vi "task_Meas.vi"() -> ()   [LabVIEW 2015]
uses:
  Framework/pdbm_test_route/UsrDefine/TaskFeedbackCmd.ctl
  Framework/pdbm_test_route/UsrDefine/TaskReqst.ctl
  <vilib>/DAQmx/read.llb/DAQmx Read (Analog 2D DBL NChan NSamp).vi
  <vilib>/DAQmx/create/channels.llb/DAQmx Create Channel (AI-Voltage-Basic).vi
  <vilib>/DAQmx/configure/timing.llb/DAQmx Timing (Sample Clock).vi
  <vilib>/DAQmx/miscellaneous.llb/DAQmx Fill In Error Info.vi
  Framework/pdbm_tasks/pdbm_tasks.lvlib
  <resource>/objmgr/daqmx.rc
  Framework/pdbm_test_route/pdbm_task_route.lvlib
panel:
  in  "Tab Control":enum32{"Scope", "Spectrum Analyzer"}(tab)
  out "dV":string="142.75 µs" caption="dV:"
  out "Scope graph":dbl[][](graph)=[[-0.0025862696478761516, 0.003794052366753585, -0.011518720468357783, 0.0025179879638276377, -0.01789904248298752, -0.010242656065431836, -0.016622978080061572, -0.008966591662505888, -0.0025862696478761516, 0.003794052366753585, 0.0025179879638276377, -0.0064144628566539935, -0.0013102052449502043, -0.011518720468357783, -0.003862334050802099, -0.008966591662505888, -0.003862334050802099, -0.0064144628566539935, -0.015346913677135626, 0.0025179879638276377, 0.0012419235609016904, -0.008966591662505888, -0.0064144628566539935, -0.008966591662505888, -0.003862334050802099, -0.003862334050802099, -0.016622978080061572, -0.010242656065431836, -0.0025862696478761516, -0.005138398453728046, -0.011518720468357783, 0.003794052366753585, -0.015346913677135626, -0.015346913677135626, 0.0025179879638276377, -0.0013102052449502043, -0.0064144628566539935, 0.003794052366753585, -0.016622978080061572, 0.0025179879638276377, -0.011518720468357783, -0.008966591662505888, -0.0025862696478761516, -0.008966591662505888, -0.0025862696478761516, -0.01279478487128373, -0.01279478487128373, -0.0013102052449502043, -0.011518720468357783, 0.003794052366753585, -0.0064144628566539935, -0.008966591662505888, -0.015346913677135626, -0.0025862696478761516, -0.003862334050802099, -0.0064144628566539935, -3.4140842024256955e-05, -0.005138398453728046, -0.011518720468357783, -0.005138398453728046, -0.007690527259579941, 0.007622245575531427, -0.007690527259579941, 0.007622245575531427, -0.0064144628566539935, -0.007690527259579941, -0.0025862696478761516, -0.0064144628566539935, -0.0064144628566539935, -0.0064144628566539935, -3.4140842024256955e-05, -0.007690527259579941, -0.01789904248298752, 0.0012419235609016904, -0.0064144628566539935, 0.003794052366753585, -0.011518720468357783, -0.003862334050802099, -0.015346913677135626, 0.003794052366753585, -0.011518720468357783, -0.007690527259579941, 0.005070116769679532, -0.0025862696478761516, -0.0013102052449502043, -0.008966591662505888, -0.003862334050802099, -0.0025862696478761516, -0.015346913677135626, -0.0064144628566539935, 0.0025179879638276377, 0.0012419235609016904, 0.003794052366753585, -0.01279478487128373, -0.016622978080061572, 0.0012419235609016904, -0.005138398453728046, 0.003794052366753585, -0.003862334050802099, -0.005138398453728046, -0.008966591662505888, -0.005138398453728046, 0.003794052366753585, 0.007622245575531427, -0.0064144628566539935, -0.008966591662505888, -0.0013102052449502043, -0.0064144628566539935, 0.014002567590161163, -0.010242656065431836, -0.010242656065431836, -0.008966591662505888, -0.016622978080061572, -0.0025862696478761516, -0.0025862696478761516, 0.005070116769679532, -0.016622978080061572, -0.0013102052449502043, -0.005138398453728046, -0.0013102052449502043, -0.0013102052449502043, 0.003794052366753585, 0.017830760798939006, -0.007690527259579941, -0.020451171288839415, -0.010242656065431836, -0.0013102052449502043, 0.005070116769679532, 0.014002567590161163, 0.007622245575531427, 0.00634618117260548, -0.011518720468357783, -0.0013102052449502043, -0.011518720468357783, -0.0025862696478761516, -0.0064144628566539935, -0.0025862696478761516, -0.0025862696478761516, 0.008898309978457374, 0.00634618117260548, -0.005138398453728046, 0.0025179879638276377, -0.008966591662505888, -0.007690527259579941, 0.005070116769679532, -0.0064144628566539935, 0.005070116769679532, -3.4140842024256955e-05, -0.005138398453728046, 0.0012419235609016904, -0.015346913677135626, 0.003794052366753585, -0.007690527259579941, 0.008898309978457374, 0.0025179879638276377, 0.0025179879638276377, -0.0013102052449502043, -3.4140842024256955e-05, 0.003794052366753585, 0.003794052366753585, -0.003862334050802099, 0.003794052366753585, -0.005138398453728046, -0.0064144628566539935, -0.008966591662505888, -0.0064144628566539935, -0.0013102052449502043, -0.007690527259579941, -3.4140842024256955e-05, -0.003862334050802099, 0.007622245575531427, 0.003794052366753585, 0.003794052366753585, -3.4140842024256955e-05, 0.003794052366753585, 0.003794052366753585, 0.008898309978457374, 0.012726503187235217, 0.0025179879638276377, -0.0025862696478761516, -0.0025862696478761516, -0.003862334050802099, -0.0013102052449502043, -0.0064144628566539935, -0.003862334050802099, 0.0025179879638276377, 0.008898309978457374, 0.005070116769679532, -0.0025862696478761516, 0.00634618117260548, 0.014002567590161163, -0.008966591662505888, 0.008898309978457374, 0.0025179879638276377, 0.014002567590161163, -0.0013102052449502043, 0.003794052366753585, -0.0025862696478761516, 0.01527863199308711, -0.005138398453728046], [-0.00392960120349739, 0.0037154429290138027, 0.0037154429290138027, -0.0013812531593269933, 0.006263790973184202, 0.0037154429290138027, 0.0037154429290138027, 0.006263790973184202, -0.00392960120349739, 0.0037154429290138027, 0.008812139017354599, -0.0013812531593269933, 0.0037154429290138027, 0.0037154429290138027, 0.0011670948848434039, 0.008812139017354599, 0.0037154429290138027, 0.0037154429290138027, 0.008812139017354599, -0.0013812531593269933, 0.0037154429290138027, 0.0037154429290138027, 0.0037154429290138027, 0.006263790973184202, -0.0013812531593269933, 0.0011670948848434039, 0.0037154429290138027, -0.0013812531593269933, 0.006263790973184202, 0.0037154429290138027, 0.0037154429290138027, 0.0011670948848434039, -0.0013812531593269933, 0.006263790973184202, 0.0037154429290138027, 0.0011670948848434039, 0.0037154429290138027, 0.0011670948848434039, 0.006263790973184202, -0.0013812531593269933, 0.0037154429290138027, 0.0011670948848434039, 0.0011670948848434039, 0.011360487061524996, -0.0013812531593269933, 0.0037154429290138027, 0.0037154429290138027, 0.0037154429290138027, 0.008812139017354599, -0.0013812531593269933, 0.011360487061524996, 0.0037154429290138027, 0.0037154429290138027, 0.0037154429290138027, -0.00392960120349739, 0.008812139017354599, -0.0013812531593269933, 0.0037154429290138027, 0.0037154429290138027, 0.0037154429290138027, 0.008812139017354599, 0.0011670948848434039, 0.006263790973184202, -0.00392960120349739, 0.0011670948848434039, 0.0011670948848434039, 0.0037154429290138027, 0.011360487061524996, -0.0013812531593269933, 0.008812139017354599, -0.0013812531593269933, 0.0037154429290138027, 0.0037154429290138027, 0.0037154429290138027, 0.0037154429290138027, -0.0013812531593269933, 0.006263790973184202, -0.0013812531593269933, 0.011360487061524996, 0.0037154429290138027, 0.0037154429290138027, 0.0011670948848434039, 0.0037154429290138027, 0.008812139017354599, -0.0013812531593269933, 0.011360487061524996, -0.006477949247667789, 0.006263790973184202, 0.0037154429290138027, 0.0037154429290138027, 0.006263790973184202, 0.0011670948848434039, 0.0011670948848434039, -0.0013812531593269933, 0.008812139017354599, -0.0013812531593269933, 0.008812139017354599, 0.0011670948848434039, 0.0037154429290138027, 0.0011670948848434039, 0.0037154429290138027, 0.0011670948848434039, 0.0037154429290138027, 0.0037154429290138027, -0.0013812531593269933, 0.008812139017354599, -0.0013812531593269933, 0.008812139017354599, -0.0013812531593269933, 0.0037154429290138027, 0.0037154429290138027, 0.0037154429290138027, 0.0037154429290138027, 0.0037154429290138027, 0.0037154429290138027, 0.0037154429290138027, 0.008812139017354599, -0.0013812531593269933, 0.006263790973184202, -0.0013812531593269933, 0.006263790973184202, 0.0011670948848434039, 0.008812139017354599, 0.0037154429290138027, 0.006263790973184202, 0.0037154429290138027, 0.0037154429290138027, 0.0037154429290138027, 0.0037154429290138027, 0.0037154429290138027, 0.006263790973184202, 0.008812139017354599, -0.0013812531593269933, 0.008812139017354599, -0.0013812531593269933, 0.006263790973184202, -0.0013812531593269933, 0.008812139017354599, 0.0011670948848434039, 0.006263790973184202, 0.0037154429290138027, 0.0037154429290138027, 0.0037154429290138027, 0.0037154429290138027, 0.0037154429290138027, 0.0037154429290138027, 0.006263790973184202, 0.0037154429290138027, 0.0037154429290138027, 0.0037154429290138027, 0.008812139017354599, -0.0013812531593269933, 0.008812139017354599, -0.0013812531593269933, 0.011360487061524996, -0.0013812531593269933, 0.008812139017354599, -0.0013812531593269933, 0.011360487061524996, -0.0013812531593269933, 0.011360487061524996, -0.0013812531593269933, 0.0037154429290138027, 0.0037154429290138027, 0.0037154429290138027, 0.0037154429290138027, 0.0037154429290138027, 0.0037154429290138027, 0.0037154429290138027, 0.0037154429290138027, 0.0037154429290138027, 0.0011670948848434039, 0.0037154429290138027, 0.0037154429290138027, 0.0037154429290138027, 0.0037154429290138027, 0.0037154429290138027, 0.0037154429290138027, 0.0037154429290138027, 0.006263790973184202, -0.0013812531593269933, 0.008812139017354599, -0.00392960120349739, 0.006263790973184202, -0.0013812531593269933, 0.006263790973184202, -0.0013812531593269933, 0.008812139017354599, -0.0013812531593269933, 0.008812139017354599, 0.0011670948848434039, 0.008812139017354599, -0.0013812531593269933, 0.011360487061524996, 0.0011670948848434039, 0.008812139017354599, 0.0011670948848434039, 0.008812139017354599, 0.0011670948848434039, 0.008812139017354599]]
  out "Ch 1 Freq":string="0 kHz" caption="Ch 1 Freq:"
  out "Ch 0 Freq":string="0 Hz" caption="Ch 0 Freq:"
  out "Ch 0 Amp":string="0 V" caption="Ch 0 Amplitude:"
  out "Ch 1 Amp":string="0 V" caption="Ch 1 Amplitude:"
  out "Acq Rate (kHz)":dbl=20.0 caption="Acq Rate:" format="%#_2g"
  out "dT":string="142.75 µs" caption="dt:"
  out "C1 Voltage":string="-4.92 V" caption="C1:"
  out "C2 Voltage":string="-4.91 V" caption="C2:"
  in  "Center Cursor":bool caption="Differential Ch 1"
  out "Ch 0 Amplitude\n(Peak to Peak)":string
  out "Ch 1 Amplitude\n(Peak to Peak)":string
  out "Freq at Cursor":string
  out "Ch 1 Main Freq":string
  out "Ch 0 Main Freq":string
  in  "X Scroll (Hz)":i32(slide)=10000 caption="X Axis Scroll" scale=10.0..50000.0 scale format="%.0p"
  in  "X Axis Zoom":i32(slide)=10000 scale=100.0..10000.0
  out "Power Spectrum":T1(graph)=[{"df"=0.0, "df"=2.0, "Power Spectrum (V^2 rms)"=array[5000 elements]}, {"df"=0.0, "df"=2.0, "Power Spectrum (V^2 rms)"=array[5000 elements]}]
  in  "Trigger Channel":u16(ring) items=["Channel 0", "Channel 1"]
  in  "Trigger Slope":bool caption="Edge"
  in  "Timebase":i32(knob)=3 caption="/div" scale=0.0..8.0
  in  "CH 0 Scale":u32(knob)=6 caption="/div" scale=0.0..8.0
  in  "CH 1 Scale":u32(knob)=6 caption="/div" scale=0.0..8.0
  in  "Level":dbl caption="V"
  in  "CH A Vert Pos":sgl(knob) caption="Position" scale=-10.0..10.0 scale format="%.1f"
  in  "CH B Vert Pos":sgl(knob) caption="Position" scale=-10.0..10.0 scale format="%.1f"
  in  "CH A Zero Pos":bool
  in  "CH B Zero Pos":bool
  in  "Reset":bool
  in  "Cursors":bool
  in  "Log":bool
  in  "C1 Select":u32(ring) caption="C1" items=["CH 0", "CH 1"]
  out "Hidden Scope":dbl[][](graph)
  in  "CH A Center":bool
  in  "CH B Center":bool
  out "Hidden Power Spectrum":T1(graph)=[{"df"=0.0, "df"=2.0, "Power Spectrum (V^2 rms)"=array[5000 elements]}, {"df"=0.0, "df"=2.0, "Power Spectrum (V^2 rms)"=array[5000 elements]}]
  in  "Device":dbl=1.0 min=1.0 max=20.0 step=1.0 format="%#_1g"
  in  "Print":bool
  in  "CH A Display":bool=TRUE caption="Differental Ch 0"
  out "Channel A LED":bool=TRUE
  in  "Stop":bool
  in  "Lock Cursors":bool
  in  "Help":bool
  out "Rate":dbl=20000.0
  in  "Input Voltage Range":u16(ring)=2 items=["1 V", "5 V", "10 V", "20 V"]
  out "Acq Rate (Hz)":dbl=20.0 caption="Acq Rate:" format="%#_2g"
  in  "error in (no error)":errorcluster
  in  "pdbm_task_data":T2
  # "kHz"
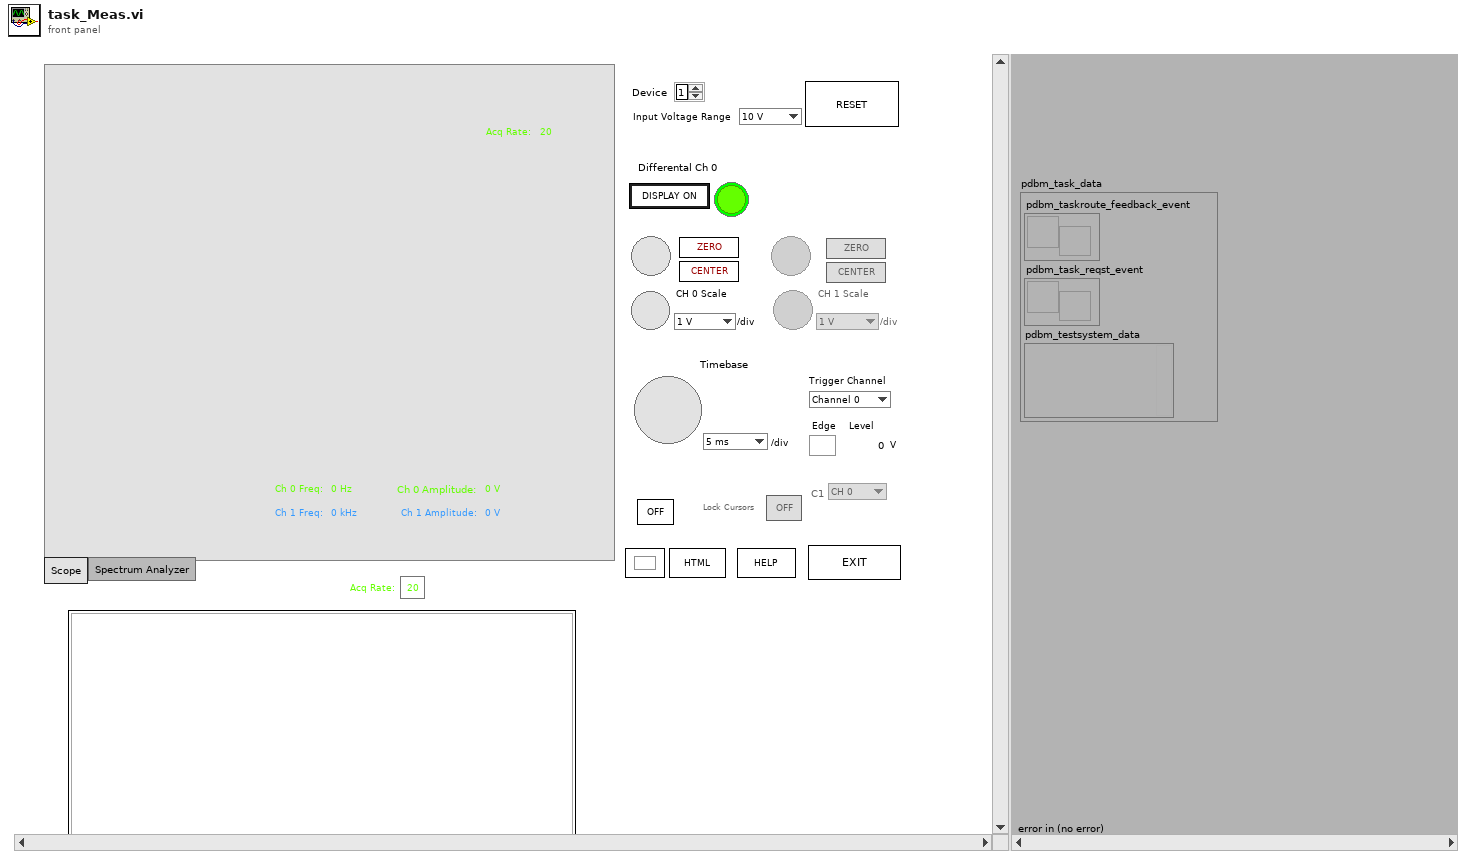
[diagram p1: front panel]
types:
  T1 = cluster{"df":dbl, "df":dbl, "Power Spectrum (V^2 rms)":dbl[]}[]
  T2 = cluster{"pdbm_taskroute_feedback_event":refnum<user-event>, "pdbm_task_reqst_event":refnum<user-event>, "pdbm_testsystem_data":variant}
  T3 = typedef "pdbm_tasks.lvlib/PDBM_TestSystem_Data.ctl" = cluster{"pdbm_general_report_info":refnum<vi>, "pdbm_task_progress":refnum<vi>, "pdbm_TestButton":refnum<vi>}
  T4 = cluster{"pdbm_task_reqst_event":refnum<user-event>, "pdbm_taskroute_feedback_event":refnum<user-event>}
  T5 = cluster{"Minimum":dbl, "Maximum":dbl, "Increment":dbl, "Minor Incr":dbl, "Start":dbl}
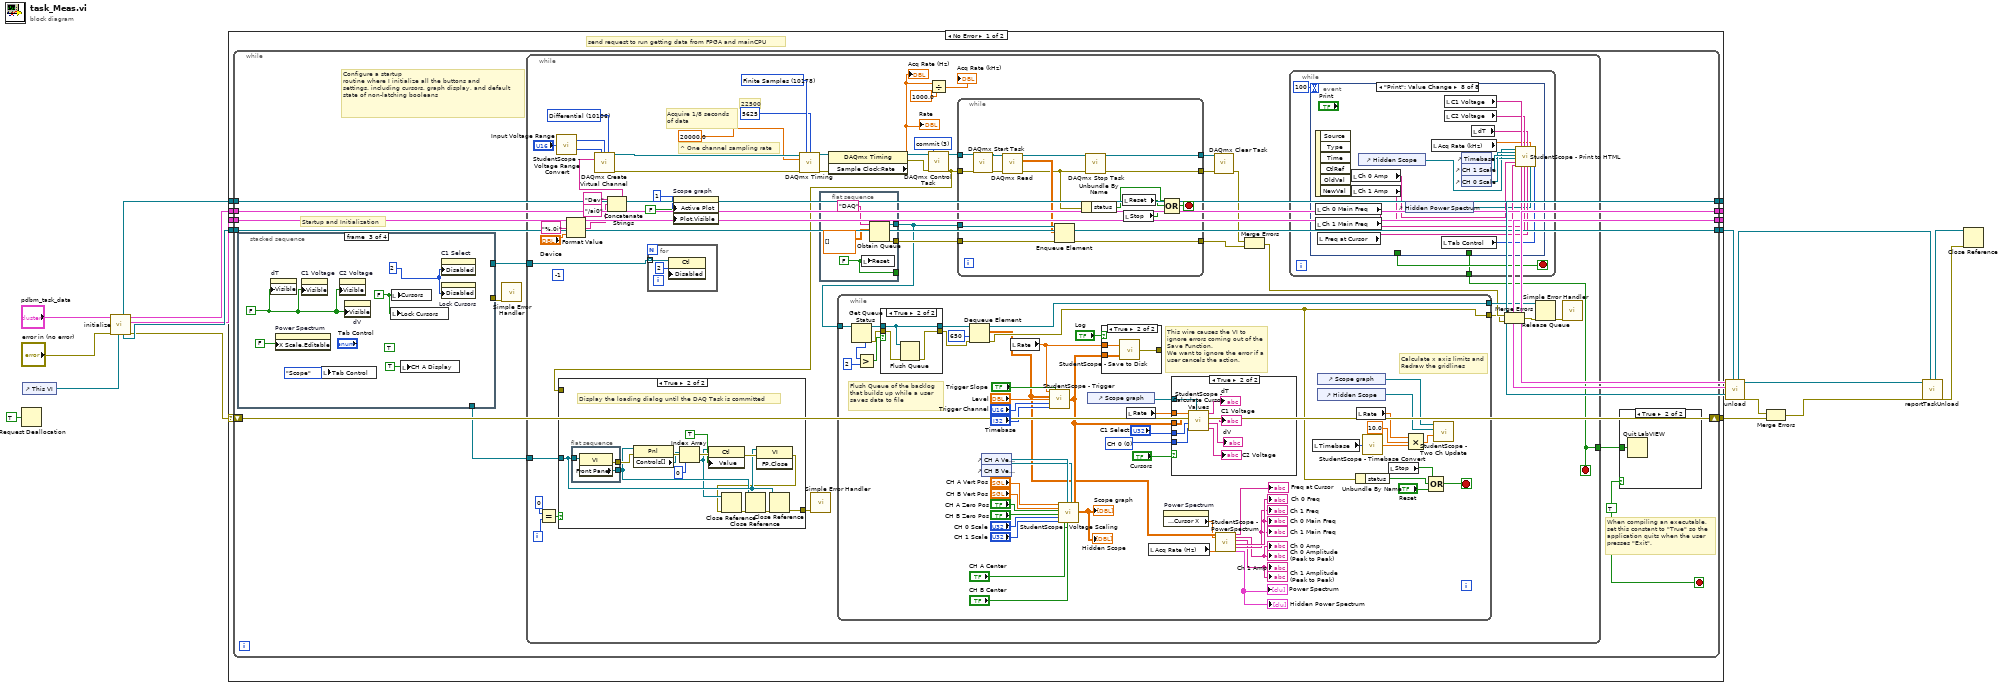
[diagram p0: block diagram]
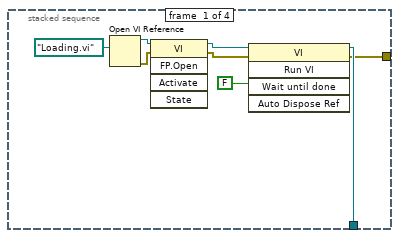
[diagram p3: hidden frame]
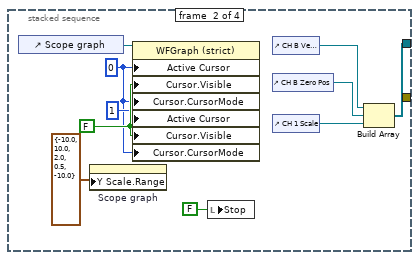
[diagram p4: hidden frame]
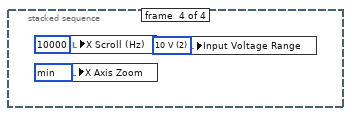
[diagram p5: hidden frame]
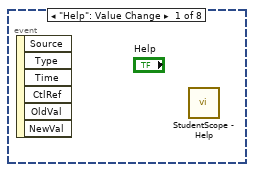
[diagram p7: hidden frame]
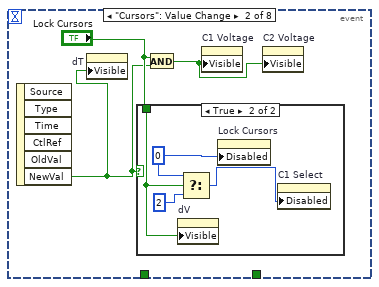
[diagram p8: hidden frame]
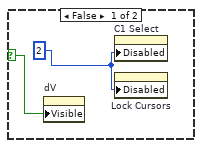
[diagram p9: hidden frame]
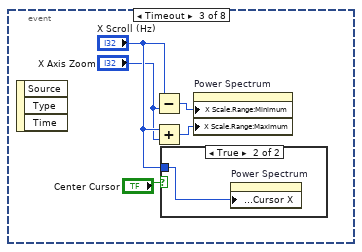
[diagram p10: hidden frame]
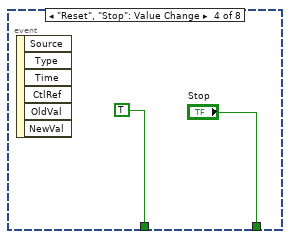
[diagram p12: hidden frame]
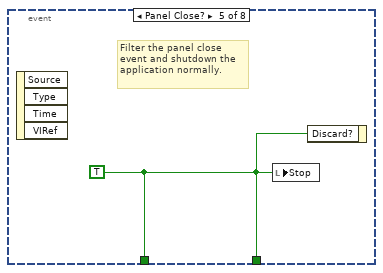
[diagram p13: hidden frame]
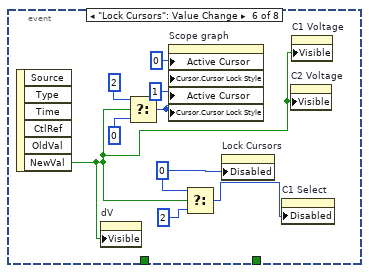
[diagram p14: hidden frame]
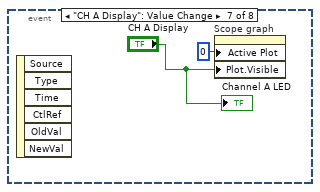
[diagram p15: hidden frame]
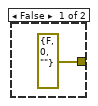
[diagram p17: hidden frame]
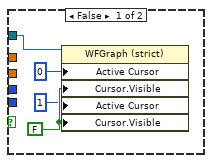
[diagram p18: hidden frame]
diagram:
  n1 = Request Deallocation(TRUE ("flag")) -> ()
  n2 = control-ref of="This VI"() -> (w19:refnum<vi>)
  n3 = call "initialize.vi"("TaskRef in"=w19, "error in"="error in (no error)", "pdbm_task_data"="pdbm_task_data") -> ("error out"=w15:errorcluster, "pdbm_task_data"=w3:T3, "pdbm_task_event"=w16:T4, "TaskRef out"=w17:refnum<vi>, "pdbm_task_reg_reqst_event"=w14:refnum<event-registration>)  [unwired: 4 in]
  n4 = case shown="No Error" w15 {
    selector: w15 -> [w29 w280]
    tunnel: w3 -> [w21 w278]
    tunnel: [w28 w280] -> w10
    tunnel: w17 -> [w23 w277]
    tunnel: w16 -> [w27 w279]
    tunnel: w14 -> [w30 w276]
    tunnel: [w26 w279] -> w13
    tunnel: [w25 w278] -> w12
    tunnel: [w24 w277] -> w2
    tunnel: [w22 w276] -> w11
    frame No Error {
      (unwired) -1
      # "send request to run getting data from FPGA and mainCPU"
      n5 = while {
        tunnel: w30 -> [w37]
        shift-right: [w36] -> w28
        shift-left: w29 -> [w36]
        tunnel: w23 -> [w38]
        tunnel: w21 -> [w39]
        tunnel: w27 -> [w40]
        tunnel: [w40] -> w26
        tunnel: [w39] -> w25
        tunnel: [w38] -> w24
        tunnel: [w37] -> w22
        stop <- w31 stop-if-true
        w31 = TRUE
        # "When compiling an executable, set this constant to \"True\" so the application quits when the user presses \"Exit\"."
        # "Startup and Initialization"
        # "Configure a startup\nroutine where I initialize all the buttons and\nsettings. including cursors, graph display, and default\nstate of non-latching booleans"
        n6 = stacked-sequence {
          tunnel: [_ w51 _ _] -> w35
          tunnel: [w43 _ _ _] -> w33
          tunnel: [w42 _ _ _] -> w34
          frame #0 {
            n7 = Open VI Reference(vi path=path "Loading.vi") -> (vi reference=w47:refnum<vi>, error out=w46:errorcluster)  [unwired: 5 in]
            n8 = invoke class="VI" method="FP.Open"(reference=w47, error in=w46) -> (reference out=w45:refnum<vi>, error out=w44:errorcluster)  [unwired: 3 in, 3 out]
            n9 = invoke class="VI" method="Run VI"(reference=w45, error in=w44, "Wait until done"=FALSE) -> (reference out=w43:refnum<vi>, error out=w42:errorcluster)  [unwired: 2 in, 3 out]
          }
          frame #1 {
            w53 = FALSE ("Cursor.Visible")
            w50 = u32 0 ("Active Cursor")
            n10 = control-ref of="Scope graph"() -> (w54:refnum<vi>)
            n11 = property on="Scope graph" class="WFGraph (strict)"("Y Scale.Range"=T5 {"Minimum"=-10.0, "Maximum"=10.0, "Increment"=2.0, "Minor Incr"=0.5, "Start"=-10.0}) -> ()  [unwired: 2 in, 2 out]
            n12 = property class="WFGraph (strict)"(reference=w54, "Active Cursor"=w50, "Cursor.Visible"=w53, "Cursor.CursorMode"=w50, "Active Cursor"=u32 1, "Cursor.Visible"=w53, "Cursor.CursorMode"=w50) -> ()  [unwired: 1 in, 2 out]
            n13 = local write "Stop"(FALSE ("stop")) -> ()
            n14 = control-ref of="CH B Vert Pos"() -> (w58:refnum<vi>)
            n15 = control-ref of="CH B Zero Pos"() -> (w57:refnum<vi>)
            n16 = control-ref of="CH 1 Scale"() -> (w56:refnum<vi>)
            n17 = Build Array(w58, w57, w56) -> (w51:refnum<vi>[])
          }
          frame #2 {
            (unwired) TRUE ("CH B Display")
            w64 = FALSE ("Cursors")
            w60 = FALSE ("Visible")
            w65 = u8 2 ("Disabled")
            n18 = property on="dT" class="Str"("Visible"=w60) -> ()  [unwired: 2 in, 2 out]
            n19 = property on="Power Spectrum" class="WFGraph (strict)"("X Scale.Editable"=FALSE) -> ()  [unwired: 2 in, 2 out]
            n20 = property on="C1 Voltage" class="Str"("Visible"=w60) -> ()  [unwired: 2 in, 2 out]
            n21 = local write "Tab Control"(enum32{"Scope", "Spectrum Analyzer"}."Scope" ("Tab Control")) -> ()
            n22 = property on="C2 Voltage" class="Str"("Visible"=w60) -> ()  [unwired: 2 in, 2 out]
            n23 = property on="dV" class="Str"("Visible"=w60) -> ()  [unwired: 2 in, 2 out]
            n24 = local write "Lock Cursors"(w64) -> ()
            n25 = local write "Cursors"(w64) -> ()
            n26 = local write "CH A Display"(TRUE ("CH B Display")) -> ()
            n27 = property on="C1 Select" class="Ring (strict)"("Disabled"=w65) -> ()  [unwired: 2 in, 2 out]
            n28 = property on="Lock Cursors" class="Bool (strict)"("Disabled"=w65) -> ()  [unwired: 2 in, 2 out]
          }
          frame #3 {
            w66 = u16 2 items=["1 V", "5 V", "10 V", "20 V"] ("Input Voltage Range")
            w67 = 10000 items=["min"=10000, ""=1000, "max"=100] ("X Axis Zoom")
            n29 = local write "X Axis Zoom"(w67) -> ()
            n30 = local write "X Scroll (Hz)"(10000 ("X Scroll (Hz)")) -> ()
            n31 = local write "Input Voltage Range"(w66) -> ()
          }
        }
        n32 = call <vilib>:"Simple Error Handler.vi"("error in (no error)"=w34) -> ()  [unwired: 4 in, 5 out]
        n33 = while {
          tunnel: w35 -> [w81]
          tunnel: w33 -> [w80]
          tunnel: [w78] -> w32
          i -> [w84]
          stop <- w78 stop-if-true
          w101 = 10178 items=["Finite Samples"=10178, "Continuous Samples"=10123, "Hardware Timed Single Point"=12522] ("sample mode")
          w108 = 3 items=["verify"=2, "reserve"=4, "commit"=3, "unreserve"=5, "abort"=6] ("action")
          w112 = 10106 items=["default"=-1, "RSE"=10083, "NRSE"=10078, "Differential"=10106, "Pseudodifferential"=12529] ("input terminal configuration")
          # "22500"
          # "^ One channel sampling rate"
          # "Acquire 1/8 seconds\nof data"
          n34 = Equal?(x=0, y=w84) -> (x = y?=w82:bool)
          n35 = call "StudentScope - Voltage Range Convert.vi"("Input Voltage Range"="Input Voltage Range") -> ("V min"=w87:i32, "V max"=w86:i32)
          n36 = Format Value(format string="%.0i", value (0)="Device") -> (output string=w95:string)  [unwired: 1 in]
          n37 = Concatenate Strings("Dev" ("string"), w95, "/ai0" ("string")) -> (w103:string)
          n38 = call-poly <vilib>:"DAQmx Create Virtual Channel.vi"("maximum value"=w86, "minimum value"=w87, "input terminal configuration"=w112, "physical channels"=w103) -> ("task out"=w113:refnum<k21>, "error out"=w100:errorcluster)  [unwired: 10 in]
          n39 = for {
            tunnel: w81 -> [w114] mode=indexing
            n40 = property class="Ctl"(reference=w114, "Disabled"=u8 2) -> ()  [unwired: 1 in, 2 out]
          }
          n41 = property on="Scope graph" class="WFGraph (strict)"("Active Plot"=u32 1, "Plot.Visible"=FALSE) -> ()  [unwired: 2 in, 2 out]
          n42 = call-poly <vilib>:"DAQmx Timing.vi"("task/channels in"=w113, "sample mode"=w101, "samples per channel"=5625, "rate"=20000.0 ("minimum value"), "error in"=w100) -> ("task out"=w102:refnum<k21>, "error out"=w91:errorcluster)  [unwired: 9 in]
          n43 = flat-sequence {
            tunnel: [w183] -> _
            tunnel: [w180] -> w92
            tunnel: [w179] -> w94
            frame #0 {
              w183 = FALSE ("stop")
              n44 = local write "Reset"(w183) -> ()
              n45 = Obtain Queue(name (unnamed)="DAQ", element data type=dbl[][] [] ("data")) -> (queue out=w180:refnum<queue>, error out=w179:errorcluster)  [unwired: 3 in, 1 out]
            }
          }
          n46 = property class="DAQmx Timing"(reference=w102, error in=w91) -> (reference out=w89:refnum<k21>, error out=w90:errorcluster, "Sample Clock:Rate"=w77:dbl)
          "Rate" <- w77
          "Acq Rate (Hz)" <- w77
          n47 = while {
            tunnel: w92 -> [w201]
            tunnel: [w216] -> w98
            tunnel: [w214] -> w73
            stop <- w218 stop-if-true
            w219 = u32 0 items=["CH 0", "CH 1"] ("C2 Select")
            # "This wire causes the VI to ignore errors coming out of the Save Function.\nWe want to ignore the error if a user cancels the action."
            # "Flush Queue of the backlog\nthat builds up while a user\nsaves data to file"
            # "Calculate x axis limits and\nRedraw the gridlines"
            n48 = Get Queue Status(queue=w201) -> (queue out=w204:refnum<queue>, error out=w199:errorcluster, # elements in queue=w200:i32)  [unwired: 2 in, 5 out]
            n49 = Greater?(x=w200, y=2) -> (0:w202:bool)
            n50 = case shown="True" w202 {
              tunnel: [w239 w242] -> w205
              tunnel: w204 -> [w239 w242]
              tunnel: w199 -> [w238 w241]
              tunnel: [w238 w240] -> w198
              frame False {
              }
              frame True {
                n51 = Flush Queue(queue=w242, error in (no error)=w241) -> (error out=w240:errorcluster)  [unwired: 2 out]
              }
            }
            n52 = Dequeue Element(queue=w205, timeout in ms (-1)=650, error in (no error)=w198) -> (queue out=w216:refnum<queue>, element=w195:dbl[][], error out=w214:errorcluster)  [unwired: 1 out]
            n53 = control-ref of="CH A Vert Pos"() -> (w227:refnum<vi>)
            n54 = control-ref of="CH B Vert Pos"() -> (w226:refnum<vi>)
            n55 = local read "Rate"() -> (w221:dbl)
            n56 = call "StudentScope - Trigger.vi"("Rate"=w221, "Trigger Slope"="Trigger Slope", "data"=w195, "Level"="Level", "Trigger Channel"="Trigger Channel", "Sec/Div"="Timebase") -> ("Array"=w196:dbl[][])  [unwired: 9 in]
            n57 = call "StudentScope - Voltage Scaling.vi"("CH A Vert Pos"="CH A Vert Pos", "CH B Vert Pos"="CH B Vert Pos", "CH A Zero Pos"="CH A Zero Pos", "CH B Zero Pos"="CH B Zero Pos", "CH A Scale"="CH 0 Scale", "CH B Scale"="CH 1 Scale", "CH A Center"="CH A Center", "Knob A Refnum"=w227, "CH B Center"="CH B Center", "Knob B Refnum"=w226, "Raw Y Values"=w196) -> ("Scaled Y Values"=→"Scope graph" →"Hidden Scope":dbl[][])  [unwired: 8 in]
            n58 = control-ref of="Scope graph"() -> (w224:refnum<vi>)
            n59 = case shown="True" "Log" {
              tunnel: w196 -> [_ w245]
              tunnel: w221 -> [_ w246]
              tunnel: [errorcluster {"status"=FALSE, "code"=0, "source"=""} ("error out") w244] -> _
              frame False {
              }
              frame True {
                n60 = call "StudentScope - Save to Disk.vi"("Y Values"=w245, "Rate"=w246) -> ("error out"=w244:errorcluster)  [unwired: 1 in]
              }
            }
            n61 = local read "Rate"() -> (w223:dbl)
            n62 = local read "Acq Rate (Hz)"() -> (w197:dbl)
            n63 = property on="Power Spectrum" class="WFGraph (strict)"() -> ("Cursor.Cursor Position:Cursor X"=w191:dbl)  [unwired: 2 in, 2 out]
            n64 = case shown="True" "Cursors" {
              tunnel: w196 -> [_ w258]
              tunnel: w224 -> [w247 w252]
              tunnel: w223 -> [_ w259]
              tunnel: "C1 Select" -> [_ w257]
              tunnel: w219 -> [_ w256]
              frame False {
                w249 = FALSE ("Cursor.Visible")
                n65 = property class="WFGraph (strict)"(reference=w247, "Active Cursor"=u32 0, "Cursor.Visible"=w249, "Active Cursor"=u32 1, "Cursor.Visible"=w249) -> ()  [unwired: 1 in, 2 out]
              }
              frame True {
                n66 = call "StudentScope - Calculate Cursor Values.vi"("Scope graph"=w252, "C2 Select"=w256, "C1 Select"=w257, "Array"=w258, "Rate"=w259) -> ("C2 Voltage"=→"C2 Voltage":string, "dV"=→"dV":string, "C1 Voltage"=→"C1 Voltage":string, "dT"=→"dT":string)  [unwired: 1 in]
              }
            }
            n67 = call "StudentScope - PowerSpectrum.vi"("data"=w195, "Cursor Position"=w191, "Acq Rate (Hz)"=w197) -> ("Cursor Freq"=→"Freq at Cursor":string, "Ch0 Amp"=→"Ch 0 Amp" →"Ch 0 Amplitude\n(Peak to Peak)":string, "Ch1 Amp"=→"Ch 1 Amp" →"Ch 1 Amplitude\n(Peak to Peak)":string, "Ch0 Freq"=→"Ch 0 Main Freq" →"Ch 0 Freq":string, "Ch1 Freq"=→"Ch 1 Main Freq" →"Ch 1 Freq":string, "Normalized Power Spectrum"=→"Power Spectrum" →"Hidden Power Spectrum":cluster{"df":dbl, "df":dbl, "Y":dbl[]}[])  [unwired: 11 in]
            n68 = local read "Timebase"() -> (w211:i32)
            n69 = control-ref of="Scope graph"() -> (w208:refnum<vi>)
            n70 = control-ref of="Hidden Scope"() -> (w187:refnum<vi>)
            n71 = Unbundle By Name(w214) -> ("status"=w213:bool)
            n72 = local read "Rate"() -> (w207:dbl)
            n73 = call "StudentScope - Timebase Convert.vi"("Sec/Div"=w211) -> ("Sec/Div"=w210:dbl)
            n74 = local read "Stop"() -> (w212:bool)
            n75 = Compound Arithmetic op=MULTIPLY(w207, 10.0 ("Rate"), w210) -> (w209:dbl)
            n76 = Compound Arithmetic op=OR(w212, w213, "Reset") -> (w218:bool)
            n77 = call "StudentScope - Two Ch Update.vi"("Samples/Graph"=w209, "scope graph ref 2"=w187, "scope graph ref"=w208) -> ()  [unwired: 9 in]
          }
          n78 = call <vilib>:"DAQmx Control Task.vi"("task/channels in"=w89, "action"=w108, "error in"=w90) -> ("task out"=w109:refnum<k21>, "error out"=w85:errorcluster)  [unwired: 11 in]
          n79 = case shown="True" w82 {
            tunnel: w85 -> [_ _]
            tunnel: w80 -> [_ w122]
            tunnel: [_ w121] -> w79
            frame False {
            }
            frame True {
              # "Display the loading dialog until the DAQ Task is committed"
              n80 = flat-sequence {
                tunnel: [w131] -> w123
                tunnel: [w130] -> w120
                tunnel: w122 -> [w129]
                frame #0 {
                  n81 = property class="VI"(reference=w129) -> (error out=w131:errorcluster, "Front Panel"=w130:refnum<vi>)  [unwired: 1 in, 1 out]
                }
              }
              n82 = property class="Pnl"(reference=w120, error in=w123) -> (error out=w127:errorcluster, "Controls[]"=w126:refnum<vi>[])  [unwired: 1 out]
              n83 = Index Array(array=w126, index=0) -> (element=w117:refnum<vi>)
              n84 = property class="Ctl"(reference=w117, error in=w127, "Value"=TRUE) -> (error out=w128:errorcluster)  [unwired: 1 out]
              n85 = invoke class="VI" method="FP.Close"(reference=w122, error in=w128) -> (error out=w116:errorcluster)  [unwired: 1 in, 2 out]
              n86 = Close Reference(reference=w117, error in (no error)=w116) -> (error out=w118:errorcluster)
              n87 = Close Reference(reference=w120, error in (no error)=w118) -> (error out=w119:errorcluster)
              n88 = Close Reference(reference=w122, error in (no error)=w119) -> (error out=w121:errorcluster)
            }
          }
          n89 = call <vilib>:"Simple Error Handler.vi"("error in (no error)"=w79) -> ()  [unwired: 4 in, 5 out]
          n90 = Divide(x=w77, y=1000.0) -> (x/y=→"Acq Rate (kHz)":dbl)
          n91 = while {
            tunnel: w109 -> [w275]
            tunnel: w85 -> [w261]
            tunnel: [w264] -> w110
            tunnel: w92 -> [w274]
            tunnel: w94 -> [w273]
            tunnel: [w272] -> w75
            tunnel: [w266] -> w111
            stop <- w271 stop-if-true
            n92 = call <vilib>:"DAQmx Start Task.vi"("task/channels in"=w275, "error in"=w261) -> ("task out"=w263:refnum<k21>, "error out"=w262:errorcluster)  [unwired: 12 in]
            n93 = call-poly <vilib>:"DAQmx Read.vi"("task/channels in"=w263, "error in"=w262) -> ("task out"=w267:refnum<k21>, "data"=w270:dbl[][], "error out"=w265:errorcluster)  [unwired: 11 in]
            n94 = Enqueue Element(queue=w274, element=w270, error in (no error)=w273) -> (error out=w272:errorcluster)  [unwired: 1 in, 2 out]
            n95 = Unbundle By Name(w265) -> ("status"=w269:bool)
            n96 = call <vilib>:"DAQmx Stop Task.vi"("task/channels in"=w267, "error in"=w265) -> ("task out"=w266:refnum<k21>, "error out"=w264:errorcluster)  [unwired: 12 in]
            n97 = local read "Reset"() -> (w268:bool)
            n98 = local read "Stop"() -> (w260:bool)
            n99 = Compound Arithmetic op=OR(w269, w268, w260) -> (w271:bool)
          }
          n100 = call <vilib>:"DAQmx Clear Task.vi"("task in"=w111, "error in"=w110) -> ("error out"=w76:errorcluster)  [unwired: 13 in]
          n101 = Merge Errors(w76, w75) -> (w74:errorcluster)
          n102 = while {
            tunnel: [w133] -> w78
            stop <- w134 stop-if-true
            n103 = event shown="[7] \"Print\": Value Change" {
              selector: _ -> [_ _ _ _ _ _ _ _]
              dyn-events: _ -> [_ _ _ _ _ _ _ _]
              timeout: u32 100 ("milliseconds to wait") -> [_ _ _ _ _ _ _ _]
              tunnel: [_ _ _ TRUE ("NewVal") w152 _ _ _] -> w134
              tunnel: [_ _ _ "Stop" w152 _ _ _] -> w133
              event "Help": Value Change {
                n104 = event-data() -> ()  [unwired: 1 in, 6 out]
                n105 = call "StudentScope - Help.vi"() -> ()  [unwired: 1 in]
              }
              event "Cursors": Value Change {
                n106 = event-data() -> ("NewVal"=w135:bool)  [unwired: 1 in, 5 out]
                n107 = property on="dT" class="Str"("Visible"=w135) -> ()  [unwired: 2 in, 2 out]
                n108 = case shown="True" w135 {
                  selector: w135 -> [w138 _]
                  tunnel: "Lock Cursors" -> [_ w140]
                  frame False {
                    w139 = u8 2 ("Disabled")
                    n109 = property on="dV" class="Str"("Visible"=w138) -> ()  [unwired: 2 in, 2 out]
                    n110 = property on="C1 Select" class="Ring (strict)"("Disabled"=w139) -> ()  [unwired: 2 in, 2 out]
                    n111 = property on="Lock Cursors" class="Bool (strict)"("Disabled"=w139) -> ()  [unwired: 2 in, 2 out]
                  }
                  frame True {
                    w141 = u8 0 ("Disabled")
                    n112 = property on="dV" class="Str"("Visible"=w140) -> ()  [unwired: 2 in, 2 out]
                    n113 = Select(t=w141, s=w140, f=u8 2) -> (s? t:f=w142:u8)
                    n114 = property on="Lock Cursors" class="Bool (strict)"("Disabled"=w141) -> ()  [unwired: 2 in, 2 out]
                    n115 = property on="C1 Select" class="Ring (strict)"("Disabled"=w142) -> ()  [unwired: 2 in, 2 out]
                  }
                }
                n116 = And(x="Lock Cursors", y=w135) -> (x .and. y?=w137:bool)
                n117 = property on="C1 Voltage" class="Str"("Visible"=w137) -> ()  [unwired: 2 in, 2 out]
                n118 = property on="C2 Voltage" class="Str"("Visible"=w137) -> ()  [unwired: 2 in, 2 out]
              }
              event Timeout {
                n119 = event-data() -> ()  [unwired: 1 in, 3 out]
                n120 = Subtract(x="X Scroll (Hz)", y="X Axis Zoom") -> (x-y=w146:i32)
                n121 = Add(x="X Scroll (Hz)", y="X Axis Zoom") -> (x+y=w145:i32)
                n122 = case shown="True" "Center Cursor" {
                  tunnel: "X Scroll (Hz)" -> [_ w149]
                  frame False {
                  }
                  frame True {
                    n123 = property on="Power Spectrum" class="WFGraph (strict)"("Cursor.Cursor Position:Cursor X"=w149) -> ()  [unwired: 2 in, 2 out]
                  }
                }
                n124 = property on="Power Spectrum" class="WFGraph (strict)"("X Scale.Range:Minimum"=w146, "X Scale.Range:Maximum"=w145) -> ()  [unwired: 2 in, 2 out]
              }
              event "Reset", "Stop": Value Change {
                n125 = event-data() -> ()  [unwired: 1 in, 6 out]
              }
              event Panel Close? {
                w152 = TRUE
                # "Filter the panel close event and shutdown the application normally."
                n126 = event-data() -> ()  [unwired: 1 in, 4 out]
                n127 = local write "Stop"(w152) -> ()
                n128 = event-data("Discard?"=w152) -> ()  [unwired: 1 in, 1 out]
              }
              event "Lock Cursors": Value Change {
                w154 = u8 0 ("Disabled")
                n129 = event-data() -> ("NewVal"=w153:bool)  [unwired: 1 in, 5 out]
                n130 = property on="dV" class="Str"("Visible"=w153) -> ()  [unwired: 2 in, 2 out]
                n131 = Select(t=u32 2 ("Active Cursor"), s=w153, f=u32 0 ("Active Cursor")) -> (s? t:f=w157:u32)
                n132 = property on="Scope graph" class="WFGraph (strict)"("Active Cursor"=u32 0, "Cursor.Cursor Lock Style"=w157, "Active Cursor"=u32 1, "Cursor.Cursor Lock Style"=w157) -> ()  [unwired: 2 in, 2 out]
                n133 = Select(t=w154, s=w153, f=u8 2) -> (s? t:f=w155:u8)
                n134 = property on="Lock Cursors" class="Bool (strict)"("Disabled"=w154) -> ()  [unwired: 2 in, 2 out]
                n135 = property on="C1 Select" class="Ring (strict)"("Disabled"=w155) -> ()  [unwired: 2 in, 2 out]
                n136 = property on="C2 Voltage" class="Str"("Visible"=w153) -> ()  [unwired: 2 in, 2 out]
                n137 = property on="C1 Voltage" class="Str"("Visible"=w153) -> ()  [unwired: 2 in, 2 out]
              }
              event "CH A Display": Value Change {
                n138 = event-data() -> ()  [unwired: 1 in, 6 out]
                n139 = property on="Scope graph" class="WFGraph (strict)"("Active Plot"=u32 0, "Plot.Visible"="CH A Display") -> ()  [unwired: 2 in, 2 out]
                "Channel A LED" <- "CH A Display"
              }
              event "Print": Value Change {
                n140 = event-data() -> ()  [unwired: 1 in, 6 out]
                n141 = local read "Ch 0 Main Freq"() -> (w170:string)
                n142 = local read "Ch 1 Main Freq"() -> (w169:string)
                n143 = local read "Freq at Cursor"() -> (w171:string)
                n144 = local read "Ch 0 Amp"() -> (w168:string)
                n145 = local read "Ch 1 Amp"() -> (w167:string)
                n146 = control-ref of="Hidden Scope"() -> (w166:refnum<vi>)
                n147 = control-ref of="Hidden Power Spectrum"() -> (w164:refnum<vi>)
                n148 = local read "Acq Rate (kHz)"() -> (w173:dbl)
                n149 = local read "Tab Control"() -> (w165:enum32{"Scope", "Spectrum Analyzer"})
                n150 = local read "C1 Voltage"() -> (w176:string)
                n151 = local read "C2 Voltage"() -> (w175:string)
                n152 = control-ref of="Timebase"() -> (w172:refnum<vi>)
                n153 = control-ref of="CH 1 Scale"() -> (w178:refnum<vi>)
                n154 = control-ref of="CH 0 Scale"() -> (w177:refnum<vi>)
                n155 = local read "dT"() -> (w174:string)
                n156 = call "StudentScope - Print to HTML.vi"("Scope graph"=w166, "CH 0 Scale"=w177, "CH 1 Scale"=w178, "Timebase"=w172, "Ch0 Amp"=w168, "Ch1 Amp"=w167, "C1"=w176, "Ch0 Freq"=w170, "C2"=w175, "Ch1 Freq"=w169, "dT"=w174, "Freq Cursor"=w171, "Acq Rate (kHz)"=w173, "Power Spectrum"=w164, "Tab Control 2"=w165) -> ()  [unwired: 5 in]
              }
            }
          }
          n157 = Merge Errors(w74, w73) -> (w72:errorcluster)
          n158 = Release Queue(queue=w98, error in (no error)=w72) -> (error out=w71:errorcluster)  [unwired: 1 in, 2 out]
          n159 = call <vilib>:"Simple Error Handler.vi"("error in (no error)"=w71) -> ()  [unwired: 4 in, 5 out]
        }
        n160 = case shown="True" w31 {
          tunnel: w32 -> [_ w41]
          frame False {
          }
          frame True {
            n161 = Quit LabVIEW(quit? (T)=w41) -> ()
          }
        }
      }
    }
    frame Error {
    }
  }
  n162 = call "unload.vi"("TaskRef in"=w2, "pdbm_task_reg_reqst_event"=w11, "pdbm_task_data"=w12, "pdbm_task_event"=w13) -> ("error out"=w9:errorcluster, "pdbm_taskroute_feedback_event"=w8:refnum<user-event>, "TaskRef out"=w1:refnum<vi>)  [unwired: 5 in]
  n163 = Merge Errors(w9, w10) -> (w7:errorcluster)
  n164 = call "reportTaskUnload.vi"("TaskRef"=w1, "error in (no error)"=w7, "pdbm_taskroute_feedback_event"=w8) -> ("error out"=w4:errorcluster, "TaskRef out"=w5:refnum<vi>)  [unwired: 6 in, 1 out]
  n165 = Close Reference(reference=w5, error in (no error)=w4) -> ()  [unwired: 1 out]
